vi "QueryMirror.vi"(8 "error in (no error)":errorcluster, 10 "Mirror":enum16{"Entrance", "Exit"}(ring), 11 "HRS_Spectrometer in":refnum<class "HRS_Spectrometer.lvclass">) -> (0 "error out":errorcluster, 3 "HRS_Spectrometer out":refnum<class "HRS_Spectrometer.lvclass">)   [LabVIEW 2023, in "Spectrometer Library.lvlib" / "HRS_Spectrometer.lvlib" / "HRS_Spectrometer.lvclass"]
uses:
  HRS_Spectrometer.lvclass
  HRS_Spectrometer.lvclass/HRS_Spectrometer.ctl
  <vilib>/addons/Tools/Unicode/UTF8 Tools.lvlib
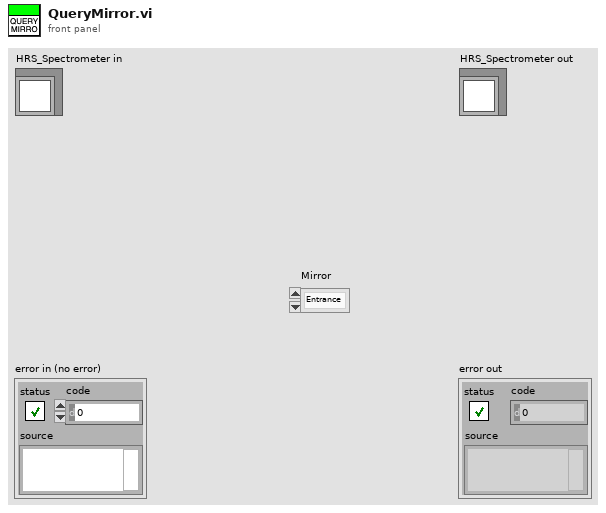
[diagram p1: front panel]
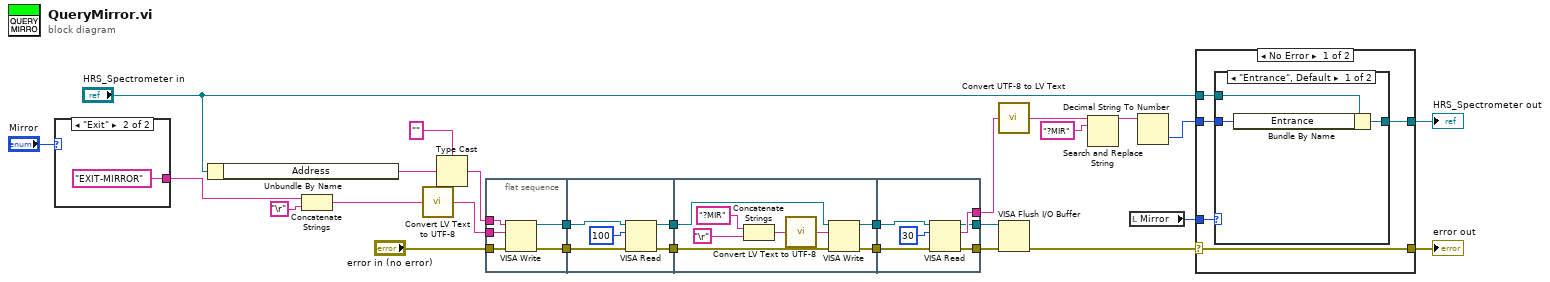
[diagram p0: block diagram]
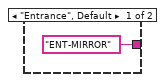
[diagram p2: hidden frame]
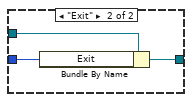
[diagram p3: hidden frame]
diagram:
  n1 = case shown="\"Exit\"" "Mirror" {
    tunnel: ["ENT-MIRROR" ("write buffer") "EXIT-MIRROR" ("write buffer")] -> w9
    frame "Entrance", Default {
    }
    frame "Exit" {
    }
  }
  n2 = Unbundle By Name("HRS_Spectrometer in") -> ("Address"=w14:string)
  n3 = Concatenate Strings(w9, "\r") -> (w8:string)
  n4 = call <vilib>:"Convert LV Text to UTF-8.vi"("LV Text"=w8) -> ("UTF-8 Text"=w12:string)  [unwired: 13 in, 1 out]
  n5 = Type Cast(type="", x=w14) -> (*(type *) &x=w13:string)
  n6 = flat-sequence {
    tunnel: [w34] -> w27
    tunnel: [w33] -> w26
    tunnel: w13 -> [w32]
    tunnel: "error in (no error)" -> [w31]
    tunnel: w12 -> [w30]
    tunnel: w27 -> [w39]
    tunnel: w26 -> [w38]
    tunnel: [w36] -> w21
    tunnel: [w37] -> w19
    tunnel: w21 -> [w47]
    tunnel: [w46] -> w20
    tunnel: w19 -> [w45]
    tunnel: [w44] -> w18
    tunnel: w20 -> [w52]
    tunnel: w18 -> [w53]
    tunnel: [w51] -> w11
    tunnel: [w50] -> w6
    tunnel: [w48] -> w7
    frame #0 {
      n7 = VISA Write(VISA resource name=w32, write buffer=w30, error in (no error)=w31) -> (VISA resource name out=w34:refnum<visa-resource-name>, error out=w33:errorcluster)  [unwired: 1 out]
    }
    frame #1 {
      n8 = VISA Read(VISA resource name=w39, byte count=u32 100, error in (no error)=w38) -> (VISA resource name out=w36:refnum<visa-resource-name>, error out=w37:errorcluster)  [unwired: 2 out]
    }
    frame #2 {
      n9 = Concatenate Strings("?MIR" ("write buffer"), "\r") -> (w40:string)
      n10 = call <vilib>:"Convert LV Text to UTF-8.vi"("LV Text"=w40) -> ("UTF-8 Text"=w43:string)  [unwired: 13 in, 1 out]
      n11 = VISA Write(VISA resource name=w47, write buffer=w43, error in (no error)=w45) -> (VISA resource name out=w46:refnum<visa-resource-name>, error out=w44:errorcluster)  [unwired: 1 out]
    }
    frame #3 {
      n12 = VISA Read(VISA resource name=w52, byte count=u32 30, error in (no error)=w53) -> (VISA resource name out=w48:refnum<visa-resource-name>, read buffer=w51:string, error out=w50:errorcluster)  [unwired: 1 out]
    }
  }
  n13 = call <vilib>:"Convert UTF-8 to LV Text.vi"("UTF-8 Text"=w11) -> ("LV Text"=w3:string)  [unwired: 13 in, 1 out]
  n14 = VISA Flush I/O Buffer(VISA resource name=w7, error in (no error)=w6) -> (error out=w5:errorcluster)  [unwired: 1 in, 1 out]
  n15 = Search and Replace String(input string=w3, search string="?MIR" ("write buffer")) -> (result string=w2:string)  [unwired: 6 in, 3 out]
  n16 = local read "Mirror"() -> (w17:enum16{"Entrance", "Exit"})
  n17 = Decimal String To Number(string=w2) -> (number=w1:i32)  [unwired: 2 in, 1 out]
  n18 = case shown="No Error" w5 {
    selector: w5 -> [w58 w66]
    tunnel: "HRS_Spectrometer in" -> [w57 w65]
    tunnel: [w58 w66] -> w16
    tunnel: [w55 w65] -> w25
    tunnel: w1 -> [w56 _]
    tunnel: w17 -> [w54 _]
    frame No Error {
      n19 = case shown="\"Entrance\", Default" w54 {
        tunnel: w57 -> [w61 w63]
        tunnel: w56 -> [w60 w62]
        tunnel: [w59 w64] -> w55
        frame "Entrance", Default {
          n20 = Bundle By Name(cluster=w61, "Entrance"=w60) -> (w59:refnum<class "HRS_Spectrometer.lvclass">)
        }
        frame "Exit" {
          n21 = Bundle By Name(cluster=w63, "Exit"=w62) -> (w64:refnum<class "HRS_Spectrometer.lvclass">)
        }
      }
    }
    frame Error {
    }
  }
  "error out" <- w16
  "HRS_Spectrometer out" <- w25
